vi "BB_Take Screenshots.vi"(8 "Error In":errorcluster, 9 "Image_Labels":string[](array[string]), 10 "Prefix":string, 11 "Image_Array":T1[](array[typedef])) -> (0 "error out":errorcluster)   [LabVIEW 2012]
uses:
  <vilib>/vision/Image Controls.llb/IMAQ Image.ctl
  <vilib>/vision/NI_Vision_Development_Module.lvlib
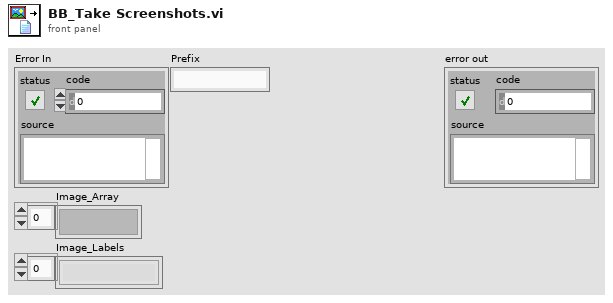
[diagram p1: front panel]
types:
  T1 = typedef "IMAQ Image.ctl" = refnum<image>
  T2 = typedef "Image Type" = u32
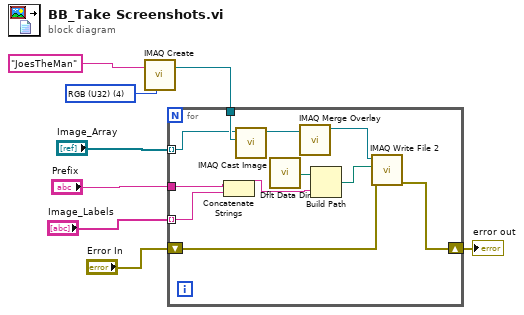
[diagram p0: block diagram]
diagram:
  w3 = T2 4 items=["Grayscale (U8)", "Grayscale (I16)", "Grayscale (SGL)", "Complex (CSG)", "RGB (U32)", "HSL (U32)", "RGB (U64)"] ("Image Type")
  n1 = call "IMAQ Create"("Image Name"="JoesTheMan", "Image Type"=w3) -> ("New Image"=w1:T1)  [unwired: 2 in, 2 out]
  n2 = for {
    tunnel: "Image_Array" -> [w9] mode=indexing
    tunnel: "Image_Labels" -> [w19] mode=indexing
    tunnel: "Prefix" -> [w18]
    shift-right: [w14] -> w8
    shift-left: "Error In" -> [w13]
    tunnel: w1 -> [w10]
    n3 = Concatenate Strings(w18, w19) -> (w15:string)
    n4 = call "IMAQ Cast Image"("Image Dst"=w10, "Image Src"=w9) -> ("Image Dst Out"=w11:T1)  [unwired: 8 in, 1 out]
    n5 = call <vilib>:"Dflt Data Dir.vi"() -> ("App:Default Data Directory"=w17:path)
    n6 = call "IMAQ Merge Overlay"("Image Src"=w11) -> ("Image Dst Out"=w12:T1)  [unwired: 9 in, 1 out]
    n7 = Build Path(base path=w17, name or relative path=w15) -> (appended path=w16:path)
    n8 = call-poly "IMAQ Write File 2"("error in (no error)"=w13, "File Path"=w16, "Image"=w12) -> ("error out"=w14:errorcluster)  [unwired: 2 in, 6 out]
  }
  "error out" <- w8
